vi "DAQ Stop.vi"(8 "error in":errorcluster, 11 "queue in":refnum<queue>) -> (0 "error out":errorcluster, 3 "queue out":refnum<queue>)   [LabVIEW 2011]
uses:
  Controls/User Event Control.ctl
  Controls/User Event Action.ctl
  Functional Global Data/Device Params Global.ctl
  Controls/User Interface Action.ctl
  Functional Global Data/Globals.ctl
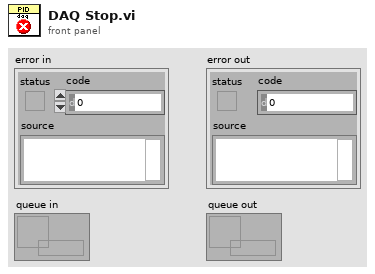
[diagram p1: front panel]
types:
  T1 = typedef "Device Params Global.ctl" = enum16{"Initialize", "Get Device Settings", "Get Device Connections", "Set Device Settings", "Set Device Connections", "Get All Device Properties"}
  T2 = typedef "User Interface Action.ctl" = enum16{"Initialize", "Data Acquisition Disable", "Data View Disable", "Sample Set", "Sample Set 2D Data", "Sample Set x0 & dx", "Sample Add", "Sample Set Cursor", "Sample Set Offset & Multiplier", "Sample Set Axis Labels", "Sample Parameters Disabled", "Sample Parameters Update", "Run Update", "Run Set Offset & Multiplier", "Run Set Axis Labels", "Run Set Cursor", "Run Set Disabled", "Run Parameters Update", "Run Parameters Disabled", "Run Number Set", "Run Number Set Range", "Run Number Set Disabled", "Sample Number Set", "Sample Number Set Range", "Notes Set Value", "Update Plot", "Set Plot Parameters", "Update Concentration Plot", "Time Set", "Clear DAQ Display", "Clear Analysis Display", "Status Bar Set", "Progress Bar Set", "Display Mode Set", "Experiment Type Set", "Analysis Plot Average Set", "Stop"}
  T3 = enum8{"Enabled", "Disabled", "Disabled and Grayed Out"}
  T4 = typedef "Globals.ctl" = enum16{"Initialize", "Get DAQ Params", "Get Data Display Params", "Set DAQ Params", "Set Data Display Params"}
  T5 = typedef "User Event Control.ctl" = cluster{"action":T6, "data":variant}
  T6 = typedef "User Event Action.ctl" = enum16{"Program Initialization", "Device Connections", "Device Settings", "Options", "DAQ Init", "PID Sample Test", "PID with PS Challenge", "PID with MFC Challenge", "Multimeter Sample Test", "Multimeter with MFC Challenge", "DAQ Stop", "Open Data File", "View Data File", "Change Display Mode", "Load INL PID Run Data", "Load Baseline-Mocon PID Data", "Load Multimeter Data", "Set Channel Sample", "Key Down", "Add Spectrum to Plot", "Add History to Plot", "Export History to Excel", "Clear Plots", "Save Plot", "Save Spectral Variable", "History Cursor Release", "Analysis Plot Cursor Release", "Program Deinitialization"}
  T7 = typedef "Data Acquisition Parameters.ctl" = cluster{"Experiment Type":T8, "Experiment Name":string, "Operator Name":string, "Notes":string, "TDMS File Path":path, "Data Acquisition State":bool, "PID Voltage Sweep":T9, "MFC Challenge Profile - Heaviside Step":T10, "MFC Challenge Profile":T11, "MFC Challenge Profile - Staircase":T12}
  T8 = typedef "DAQ Type.ctl" = enum16{"PID Sample", "PID with PS Challenge", "PID with MFC Challenge", "Multimeter Sample", "Multimeter with MFC Challenge"}
  T9 = typedef "PID Voltage Seep Settings.ctl" = cluster{"Voltage Step (V)":dbl, "Voltage Range (V)":cluster{u16, u16}, "Time Step (s)":dbl, "Voltage Step Direction":enum16{"High 2 Low", "Low 2 High"}}
  T10 = typedef "MFC Challenge Profile - Heaviside Step.ctl" = cluster{"Valve Open Duration":u16, "MFC Flow Rate":dbl, "Valve Open Repeats":u16, "Valve Open Start":u16}
  T11 = typedef "MFC Challen Profile Type.ctl" = enum16{"Heaviside", "Staircase"}
  T12 = typedef "MFC Challenge Profile - Staircase.ctl" = cluster{"Step Time Duration":u16, "Step Flow Rate":dbl, "Steps":u16, "Valve Open Start":u16, "Recovery":bool, "Repeats":u16}
  T13 = typedef "Device Connections.ctl" = cluster{"Detector":cluster{"Detector Type":T14, "Connection":bool, "B-M PID":T15, "INL PID Connections":T16}, "Power Supply":cluster{"Type":enum16{"Stanford Research PS350", "Keithley 2400"}, "Connection":bool, "VISA resource name":refnum<visa-resource-name>}, "Mass Flow Controller":cluster{"Type":enum16{"Aalborg GFC17"}, "Connection":bool, "Aalborg GFC17":T18}, "Valve Controller":cluster{"Type":T19, "Connection":bool, "SMC - INL":cluster{"VISA resource name":refnum<visa-resource-name>}}, "Multimeter":cluster{"Multimeter Type":T20, "Connection":bool, "VISA resource name":refnum<visa-resource-name>}, "Vapour Generator":cluster{"Type":T21, "Connection":bool, "Owlstone Gen-SYS":T22}}
  T14 = typedef "Detector Type.ctl" = enum16{"INL PID", "Baseline-Mocon piD-TECH plus"}
  T15 = typedef "Baseline Mocon piD-Tech plus.lvclass/Connections.ctl" = cluster{"AI DAQmx channel":tag}
  T16 = typedef "INL PID Connections.ctl" = cluster{"PIDs":u8, "Integrator DAQ Channels 1":T17, "Integrator DAQ Channels 2":T17}
  T17 = typedef "INL PID.lvclass/Integrator DAQmx Channels.ctl" = cluster{"V0":tag, "S1":tag, "S2":tag}
  T18 = typedef "Aalborg GFC17.lvclass/Aalborg GFC17 Connections.ctl" = cluster{"flow rate setpoint channel":tag, "flow rate reading channel":tag, "valve channel":tag}
  T19 = typedef "Valve Type.ctl" = enum16{"SMC - INL"}
  T20 = typedef "Multimeter Type.ctl" = enum16{"Agilent 3458A"}
  T21 = typedef "Vapour Generator Type.ctl" = enum16{"Owlstone GEN-SYS"}
  T22 = typedef "Owlstone GEN-SYS.lvclass/GEN-SYS Connections.ctl" = cluster{"GEN-SYS VISA resource name":refnum<visa-resource-name>, "OVG-4":cluster{"Flow Address":u8, "Temp Address":u8}, "OHG-4":cluster{"Flow Address":u8, "Easydew VISA resource name":refnum<visa-resource-name>}}
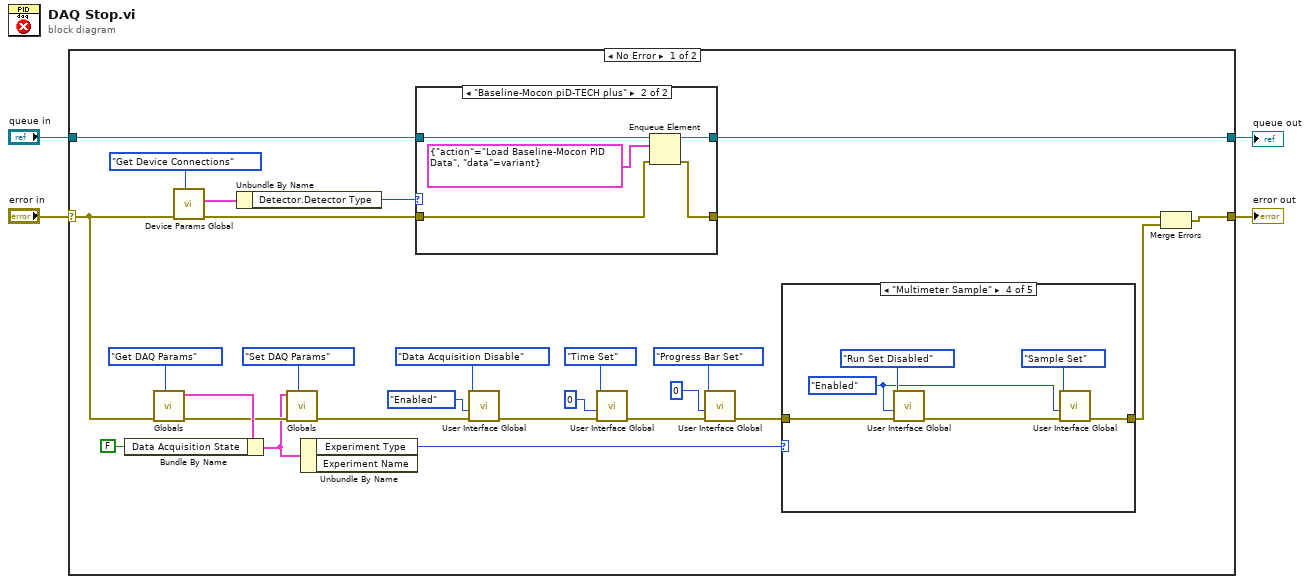
[diagram p0: block diagram]
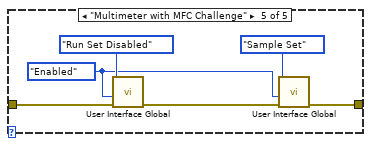
[diagram p6: hidden frame]
diagram:
  n1 = case shown="No Error" "error in" {
    selector: "error in" -> [w12 w55]
    tunnel: [w7 w55] -> w4
    tunnel: "queue in" -> [w10 w54]
    tunnel: [w5 w54] -> w1
    frame No Error {
      n2 = call "Globals.vi"("action"=Globals."Get DAQ Params", "error in"=w12) -> ("error out"=w28:errorcluster, "Data Acquisition"=w29:T7)  [unwired: 7 in, 1 out]
      n3 = Bundle By Name(cluster=w29, "Data Acquisition State"=FALSE) -> (w23:T7)
      n4 = call "Device Params Global.vi"("action"=Device_Params_Global."Get Device Connections", "error in"=w12) -> ("error out"=w9:errorcluster, "Device Connections OUT"=w13:T13)  [unwired: 7 in, 1 out]
      n5 = Unbundle By Name(w13) -> ("Detector.Detector Type"=w11:T14)
      n6 = call "Globals.vi"("action"=Globals."Set DAQ Params", "error in"=w28, "Data Acquisition"=w23) -> ("error out"=w22:errorcluster)  [unwired: 6 in, 2 out]
      n7 = Unbundle By Name(w23) -> ("Experiment Type"=w19:T8)  [unwired: 1 out]
      n8 = case shown="\"Baseline-Mocon piD-TECH plus\"" w11 {
        tunnel: w10 -> [w33 w37]
        tunnel: [w33 w36] -> w5
        tunnel: w9 -> [w32 w35]
        tunnel: [w32 w34] -> w8
        frame "INL PID", Default {
        }
        frame "Baseline-Mocon piD-TECH plus" {
          n9 = Enqueue Element(queue=w37, element=T5 {"action"=enum."Load Baseline-Mocon PID Data", "data"=variant} ("user event control"), error in (no error)=w35) -> (queue out=w36:refnum<queue>, error out=w34:errorcluster)  [unwired: 1 in, 1 out]
        }
      }
      n10 = call "User Interface Global.vi"("error in"=w22, "data1"=T3."Enabled" ("Disabled"), "action"=User_Interface_Action."Data Acquisition Disable" ("Action")) -> ("error out"=w25:errorcluster)  [unwired: 8 in]
      n11 = call "User Interface Global.vi"("error in"=w25, "data1"=0, "action"=User_Interface_Action."Time Set") -> ("error out"=w15:errorcluster)  [unwired: 8 in]
      n12 = call "User Interface Global.vi"("error in"=w15, "data1"=u8 0, "action"=User_Interface_Action."Progress Bar Set") -> ("error out"=w16:errorcluster)  [unwired: 8 in]
      n13 = case shown="\"Multimeter Sample\"" w19 {
        tunnel: w16 -> [w39 w40 w41 w42 w49]
        tunnel: [w39 w40 w41 w44 w48] -> w6
        frame "PID Sample", Default {
        }
        frame "PID with PS Challenge" {
        }
        frame "PID with MFC Challenge" {
        }
        frame "Multimeter Sample" {
          w43 = T3."Enabled" ("Disabled")
          n14 = call "User Interface Global.vi"("error in"=w42, "data1"=w43, "action"=User_Interface_Action."Run Set Disabled" ("Action")) -> ("error out"=w45:errorcluster)  [unwired: 8 in]
          n15 = call "User Interface Global.vi"("error in"=w45, "data1"=w43, "action"=User_Interface_Action."Sample Set" ("Action")) -> ("error out"=w44:errorcluster)  [unwired: 8 in]
        }
        frame "Multimeter with MFC Challenge" {
          w50 = T3."Enabled" ("Disabled")
          n16 = call "User Interface Global.vi"("error in"=w49, "data1"=w50, "action"=User_Interface_Action."Run Set Disabled" ("Action")) -> ("error out"=w51:errorcluster)  [unwired: 8 in]
          n17 = call "User Interface Global.vi"("error in"=w51, "data1"=w50, "action"=User_Interface_Action."Sample Set" ("Action")) -> ("error out"=w48:errorcluster)  [unwired: 8 in]
        }
      }
      n18 = Merge Errors(w8, w6) -> (w7:errorcluster)
    }
    frame Error {
    }
  }
  "error out" <- w4
  "queue out" <- w1
